vi "Send Packet.vi"(6 "error in (no error) 2":errorcluster, 7 "?":T2, 8 "Log string 2":string, 9 "SerialPortRef 2":T1) -> (0 "error out 2":errorcluster, 3 "SerialPortRef out 2":T1)   [LabVIEW 2016]
uses:
  <vilib>/Rock Robotics/WPI/SerialPort/WPI_SerialPortRef.ctl
  Packet Types.ctl
panel:
  in  "?":T2
  out "Sent string":string
  out "error out":errorcluster
  in  "error in (no error)":errorcluster
  out "SerialPortRef out":T1
  in  "SerialPortRef":T1
  in  "Log string":string
  # "Type:"
  # "Cannot contain line breaks or the character 0x00"
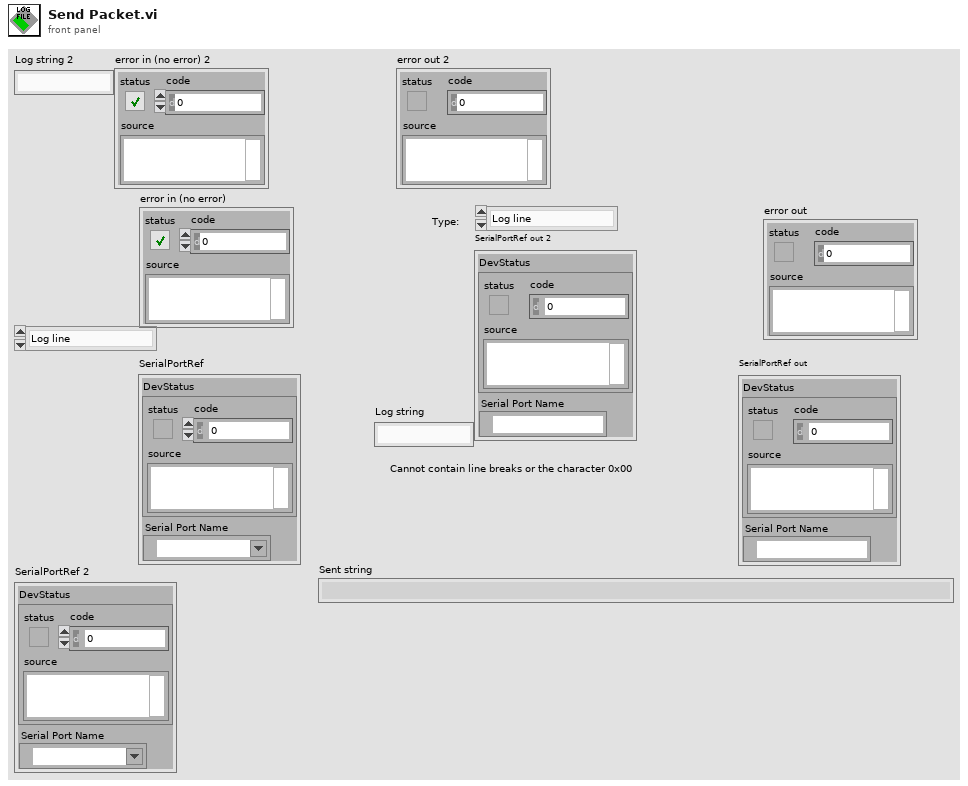
[diagram p1: front panel]
types:
  T1 = typedef "WPI_SerialPortRef.ctl" = cluster{"DevStatus":errorcluster, "Serial Port Name":refnum<visa-resource-name>}
  T2 = typedef "Packet Types.ctl" = enum16{"Log line", "Open File", "Send Header", "Set Time", "Send to LCD", "Close File"}
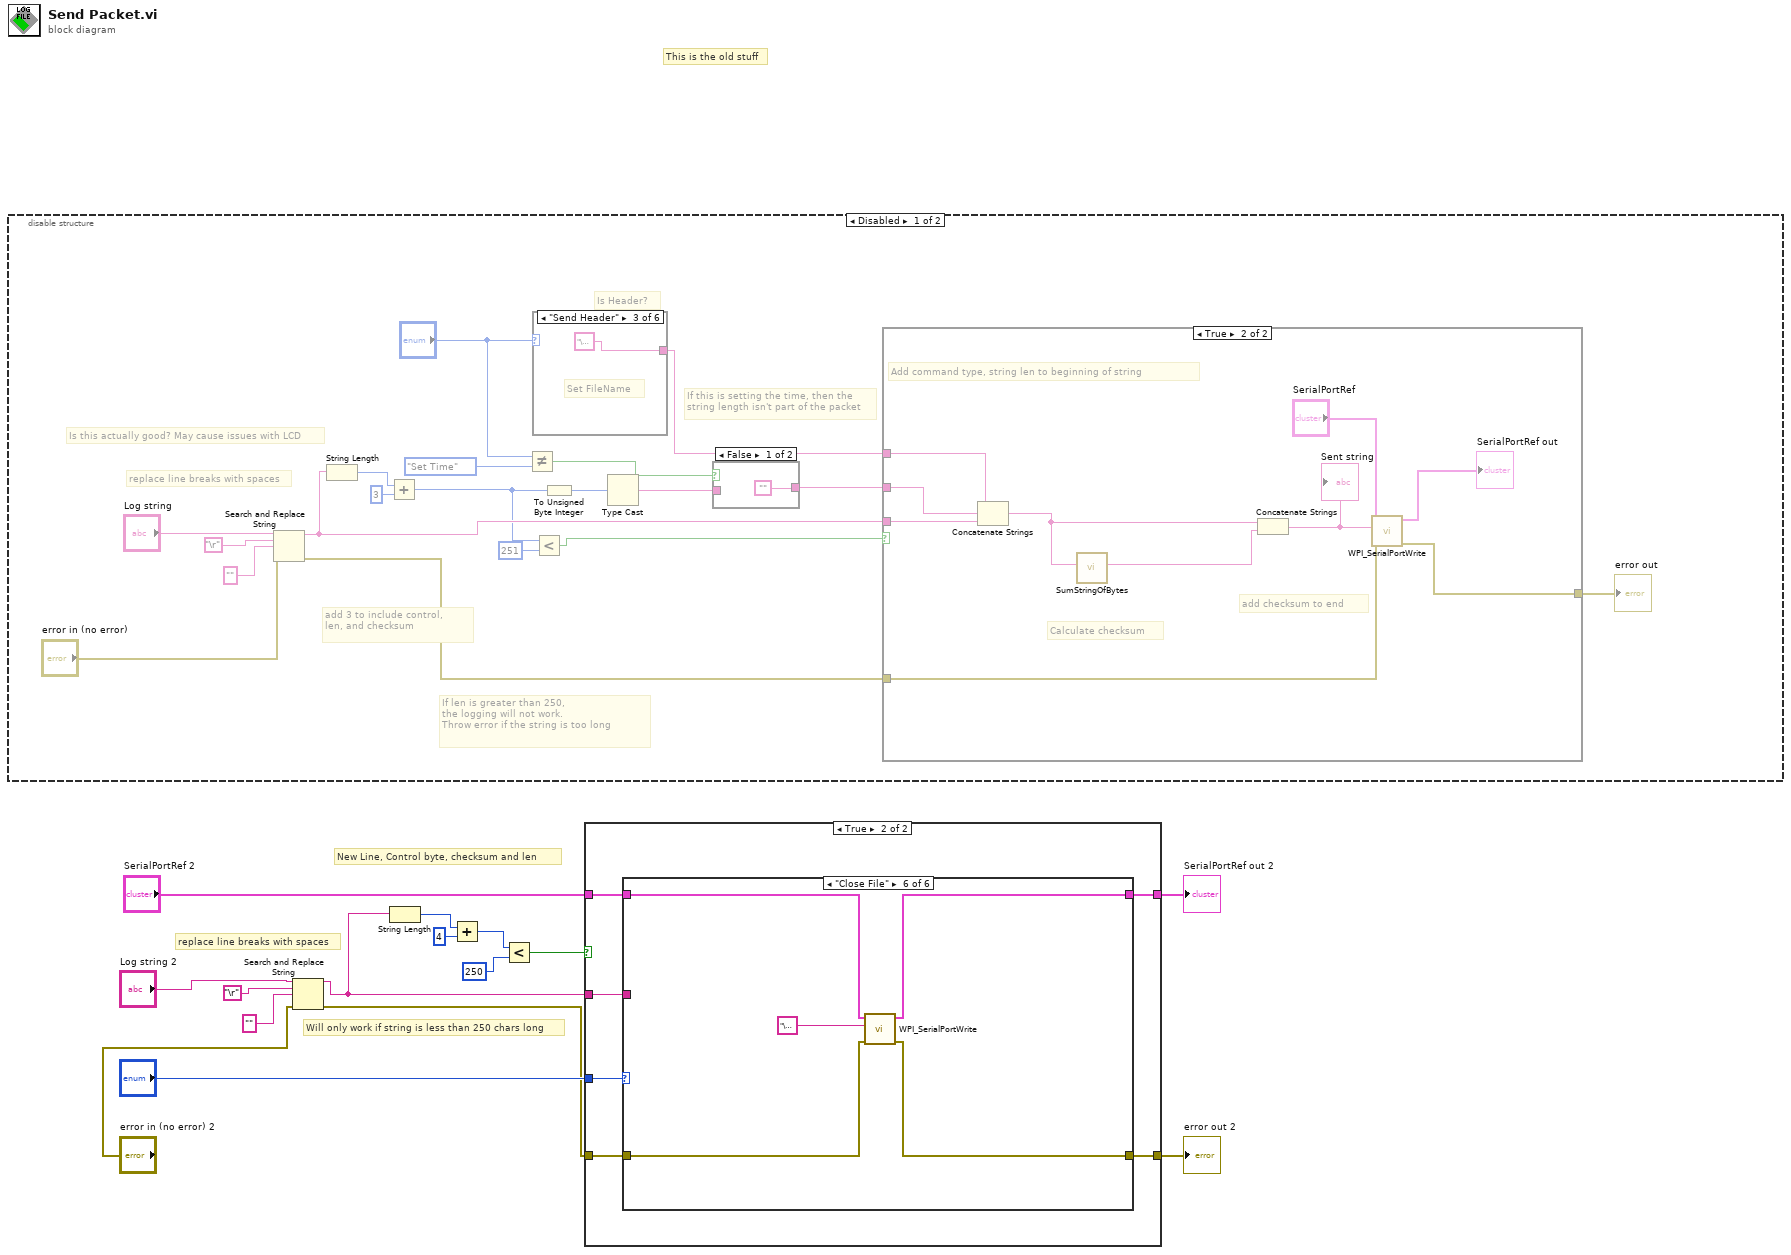
[diagram p0: block diagram]
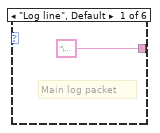
[diagram p3: hidden frame]
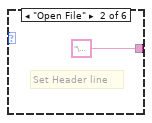
[diagram p4: hidden frame]
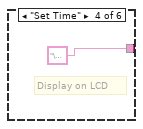
[diagram p5: hidden frame]
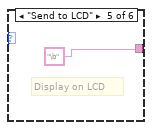
[diagram p6: hidden frame]
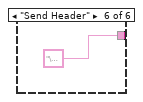
[diagram p7: hidden frame]
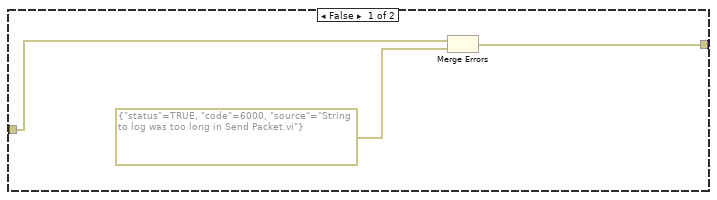
[diagram p8: hidden frame]
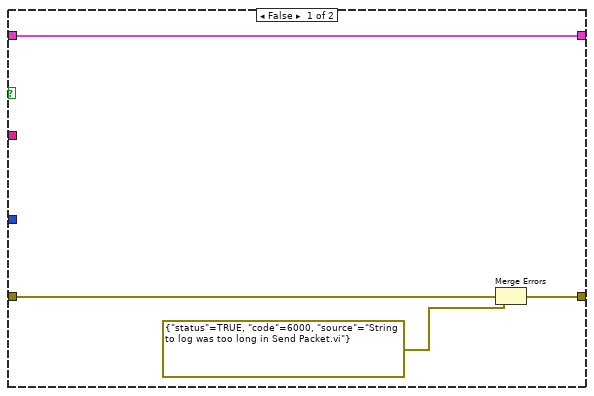
[diagram p10: hidden frame]
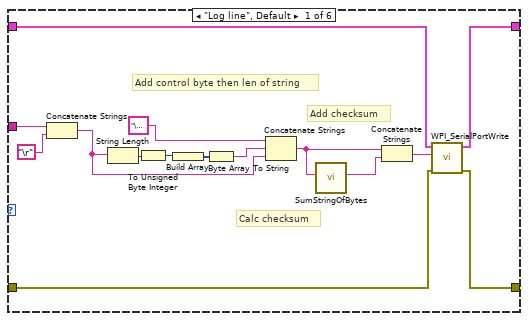
[diagram p11: hidden frame]
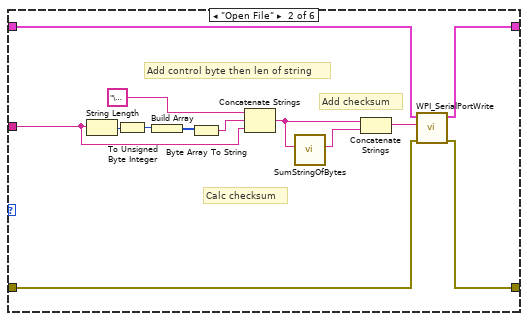
[diagram p12: hidden frame]
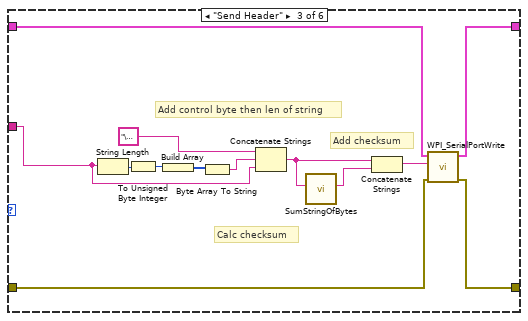
[diagram p13: hidden frame]
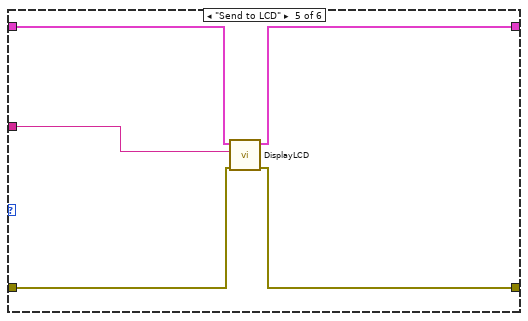
[diagram p15: hidden frame]
diagram:
  # "This is the old stuff"
  # "New Line, Control byte, checksum and len"
  # "Will only work if string is less than 250 chars long"
  # "replace line breaks with spaces"
  n1 = disable-structure shown="Disabled" {
    frame Disabled {
      # "If this is setting the time, then the \nstring length isn't part of the packet"
      # "Is this actually good? May cause issues with LCD"
      # "Is Header?"
      # "If len is greater than 250,\nthe logging will not work.\nThrow error if the string is too long"
      # "add 3 to include control, \nlen, and checksum"
      # "replace line breaks with spaces"
      n2 = Search and Replace String(input string="Log string", search string="\r", replace string="" ("replace string (\"\")"), error in="error in (no error)") -> (result string=w27:string, error out=w30:errorcluster)  [unwired: 4 in, 2 out]
      n3 = String Length(string=w27) -> (length=w29:i32)
      n4 = Add(x=w29, y=3) -> (x+y=w21:i32)
      n5 = Not Equal?(x="?", y=Packet_Types."Set Time") -> (x != y?=w16:bool)
      n6 = case shown="\"Send Header\"" "?" {
        tunnel: ["\u0001" ("string") "\u0003" ("string") "\u0002" ("string") "\u0005" ("string") "\b" ("string") "\u0004" ("string")] -> w23
        frame "Log line", Default {
          # "Main log packet"
        }
        frame "Open File" {
          # "Set Header line"
        }
        frame "Send Header" {
          # "Set FileName"
        }
        frame "Set Time" {
          # "Display on LCD"
        }
        frame "Send to LCD" {
          # "Display on LCD"
        }
        frame "Send Header" {
        }
      }
      n7 = Less?(x=w21, y=251) -> (x < y?=w24:bool)
      n8 = To Unsigned Byte Integer(number=w21) -> (unsigned 8bit integer=w22:u8)
      n9 = Type Cast(x=w22) -> (*(type *) &x=w20:string)  [unwired: 1 in]
      n10 = case shown="False" w16 {
        tunnel: w20 -> [_ w36]
        tunnel: ["" w36] -> w19
        frame False {
        }
        frame True {
        }
      }
      n11 = case shown="True" w24 {
        tunnel: w30 -> [w45 w53]
        tunnel: w23 -> [_ w52]
        tunnel: w19 -> [_ w46]
        tunnel: w27 -> [_ w48]
        tunnel: [w43 w47] -> w26
        frame False {
          n12 = Merge Errors(w45, errorcluster {"status"=TRUE, "code"=6000, "source"="String to log was too long in Send Packet.vi"} ("error out")) -> (w43:errorcluster)
        }
        frame True {
          # "add checksum to end"
          # "Add command type, string len to beginning of string"
          # "Calculate checksum"
          n13 = Concatenate Strings(w52, w46, w48) -> (w51:string)
          n14 = call "SumStringOfBytes.vi"("String Of Bytes"=w51) -> ("SumAsString"=w50:string)  [unwired: 10 in]
          n15 = Concatenate Strings(w51, w50) -> (w49:string)
          "Sent string" <- w49
          n16 = call <vilib>:"WPI_SerialPortWrite.vi"("error in (no error)"=w53, "Buffer"=w49, "SerialPortRef"="SerialPortRef") -> ("error out"=w47:errorcluster, "SerialPortRef"=→"SerialPortRef out":T1)  [unwired: 6 in, 1 out]
        }
      }
      "error out" <- w26
    }
    frame Enabled {
    }
  }
  n17 = Search and Replace String(input string="Log string 2", search string="\r", replace string="" ("replace string (\"\")"), error in="error in (no error) 2") -> (result string=w4:string, error out=w1:errorcluster)  [unwired: 4 in, 2 out]
  n18 = String Length(string=w4) -> (length=w8:i32)
  n19 = Add(x=w8, y=4) -> (x+y=w6:i32)
  n20 = Less?(x=w6, y=250) -> (x < y?=w3:bool)
  n21 = case shown="True" w3 {
    tunnel: "?" -> [_ w65]
    tunnel: "SerialPortRef 2" -> [w56 w64]
    tunnel: w1 -> [w58 w63]
    tunnel: w4 -> [_ w62]
    tunnel: [w56 w61] -> w10
    tunnel: [w57 w60] -> w9
    frame False {
      n22 = Merge Errors(errorcluster {"status"=TRUE, "code"=6000, "source"="String to log was too long in Send Packet.vi"} ("error out"), w58) -> (w57:errorcluster)
    }
    frame True {
      n23 = case shown="\"Close File\"" w65 {
        tunnel: w63 -> [w73 w84 w97 w107 w111 w117]
        tunnel: w64 -> [w74 w85 w94 w108 w113 w114]
        tunnel: w62 -> [w67 w86 w95 _ w109 _]
        tunnel: [w71 w83 w98 w108 w112 w115] -> w61
        tunnel: [w72 w82 w96 w107 w110 w116] -> w60
        frame "Log line", Default {
          # "Add checksum"
          # "Add control byte then len of string"
          # "Calc checksum"
          n24 = Concatenate Strings(w67, "\r") -> (w68:string)
          n25 = String Length(string=w68) -> (length=w70:i32)
          n26 = To Unsigned Byte Integer(number=w70) -> (unsigned 8bit integer=w69:u8)
          n27 = Build Array(w69) -> (w80:u8[])
          n28 = Byte Array To String(unsigned byte array=w80) -> (string=w79:string)
          n29 = Concatenate Strings("\u0001", w79, w68) -> (w76:string)
          n30 = call "SumStringOfBytes.vi"("String Of Bytes"=w76) -> ("SumAsString"=w77:string)  [unwired: 10 in]
          n31 = Concatenate Strings(w76, w77) -> (w75:string)
          n32 = call <vilib>:"WPI_SerialPortWrite.vi"("error in (no error)"=w73, "Buffer"=w75, "SerialPortRef"=w74) -> ("error out"=w72:errorcluster, "SerialPortRef"=w71:T1)  [unwired: 6 in, 1 out]
        }
        frame "Open File" {
          # "Calc checksum"
          # "Add checksum"
          # "Add control byte then len of string"
          n33 = String Length(string=w86) -> (length=w87:i32)
          n34 = To Unsigned Byte Integer(number=w87) -> (unsigned 8bit integer=w90:u8)
          n35 = Build Array(w90) -> (w89:u8[])
          n36 = Byte Array To String(unsigned byte array=w89) -> (string=w88:string)
          n37 = Concatenate Strings("\u0003", w88, w86) -> (w92:string)
          n38 = call "SumStringOfBytes.vi"("String Of Bytes"=w92) -> ("SumAsString"=w93:string)  [unwired: 10 in]
          n39 = Concatenate Strings(w92, w93) -> (w81:string)
          n40 = call <vilib>:"WPI_SerialPortWrite.vi"("error in (no error)"=w84, "Buffer"=w81, "SerialPortRef"=w85) -> ("error out"=w82:errorcluster, "SerialPortRef"=w83:T1)  [unwired: 6 in, 1 out]
        }
        frame "Send Header" {
          # "Calc checksum"
          # "Add checksum"
          # "Add control byte then len of string"
          n41 = String Length(string=w95) -> (length=w105:i32)
          n42 = To Unsigned Byte Integer(number=w105) -> (unsigned 8bit integer=w102:u8)
          n43 = Build Array(w102) -> (w103:u8[])
          n44 = Byte Array To String(unsigned byte array=w103) -> (string=w104:string)
          n45 = Concatenate Strings("\u0002", w104, w95) -> (w100:string)
          n46 = call "SumStringOfBytes.vi"("String Of Bytes"=w100) -> ("SumAsString"=w99:string)  [unwired: 10 in]
          n47 = Concatenate Strings(w100, w99) -> (w106:string)
          n48 = call <vilib>:"WPI_SerialPortWrite.vi"("error in (no error)"=w97, "Buffer"=w106, "SerialPortRef"=w94) -> ("error out"=w96:errorcluster, "SerialPortRef"=w98:T1)  [unwired: 6 in, 1 out]
        }
        frame "Set Time" {
        }
        frame "Send to LCD" {
          n49 = call "DisplayLCD.vi"("error in (no error)"=w111, "Display string"=w109, "SerialPortRef"=w113) -> ("error out"=w110:errorcluster, "SerialPortRef 2"=w112:T1)  [unwired: 7 in]
        }
        frame "Close File" {
          n50 = call <vilib>:"WPI_SerialPortWrite.vi"("error in (no error)"=w117, "Buffer"="\u0004", "SerialPortRef"=w114) -> ("error out"=w116:errorcluster, "SerialPortRef"=w115:T1)  [unwired: 6 in, 1 out]
        }
      }
    }
  }
  "SerialPortRef out 2" <- w10
  "error out 2" <- w9
